vi "Is Naughty Func.vi"(10 "GObj Refnum":refnum<vi>) -> (1 "Function":string, 2 "Naughty Function":bool, 5 "Is Func":bool)   [LabVIEW 2024, in "Word Search Scorer.lvlib"]
uses:
  Word Search Scorer.lvlib
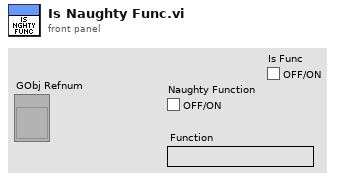
[diagram p1: front panel]
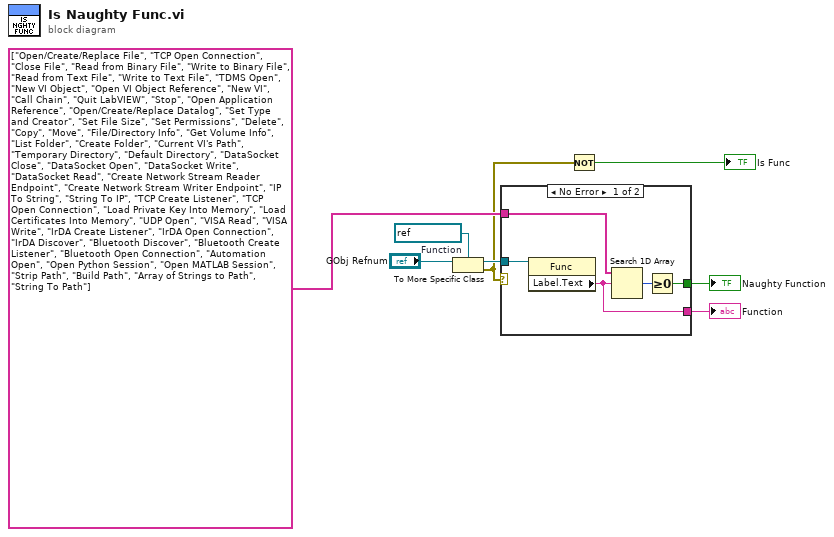
[diagram p0: block diagram]
diagram:
  w4 = refnum<vi> refnum  # Function
  n1 = To More Specific Class(target class=w4, reference="GObj Refnum") -> (specific class reference=w5:refnum<vi>, error out=w2:errorcluster)  [unwired: 1 in]
  n2 = case shown="No Error" w2 {
    tunnel: string[] ["Open/Create/Replace File", "TCP Open Connection", "Close File", "Read from Binary File", "Write to Binary File", "Read from Text File", "Write to Text File", "TDMS Open", "New VI Object", "Open VI Object Reference", "New VI", "Call Chain", "Quit LabVIEW", "Stop", "Open Application Reference", "Open/Create/Replace Datalog", "Set Type and Creator", "Set File Size", "Set Permissions", "Delete", "Copy", "Move", "File/Directory Info", "Get Volume Info", "List Folder", "Create Folder", "Current VI's Path", "Temporary Directory", "Default Directory", "DataSocket Close", "DataSocket Open", "DataSocket Write", "DataSocket Read", "Create Network Stream Reader Endpoint", "Create Network Stream Writer Endpoint", "IP To String", "String To IP", "TCP Create Listener", "TCP Open Connection", "Load Private Key Into Memory", "Load Certificates Into Memory", "UDP Open", "VISA Read", "VISA Write", "IrDA Create Listener", "IrDA Open Connection", "IrDA Discover", "Bluetooth Discover", "Bluetooth Create Listener", "Bluetooth Open Connection", "Automation Open", "Open Python Session", "Open MATLAB Session", "Strip Path", "Build Path", "Array of Strings to Path", "String To Path"] -> [w13 _]
    tunnel: [w11 _] -> w7
    tunnel: w5 -> [w10 _]
    tunnel: [w9 _] -> w3
    frame No Error {
      n3 = property class="Func"(reference=w10) -> ("Label.Text"=w9:string)  [unwired: 1 in, 2 out]
      n4 = Search 1D Array(1D array=w13, element=w9) -> (index of element=w12:i32)  [unwired: 1 in]
      n5 = Greater Or Equal To 0?(x=w12) -> (x >= 0?=w11:bool)
    }
    frame Error {
    }
  }
  "Naughty Function" <- w7
  "Function" <- w3
  n6 = Not(x=w2) -> (.not. x?=→"Is Func":bool)
